vi "Update Channel UI.vi"(8 "error in (no error)":errorcluster, 10 "Channels":T1[][](array[typedef]), 11 "CIF_UI in":refnum<class "CIF_UI.lvclass">) -> (0 "error out":errorcluster, 3 "CIF_UI out":refnum<class "CIF_UI.lvclass">)   [LabVIEW 2021, in "CIF_UI.lvclass"]
uses:
  CIF_UI.lvclass
  CIFCore/Grpc/CIFCoreChannel_client/RPC Messages/cif_channelcore_Channel.ctl
  CIFCore/Grpc/CIFCoreChannel_client/RPC Messages/cif_channelcore_Direction.ctl
  CIFCore/Grpc/CIFCoreChannel_client/RPC Messages/cif_channelcore_PATTERN.ctl
  CIF_UI.lvclass/CIF_UI.ctl
  Typedef/Direction to Include.ctl
  CIFCore/Grpc/CIFCoreChannel_client/CIFCoreChannel_client.lvlib
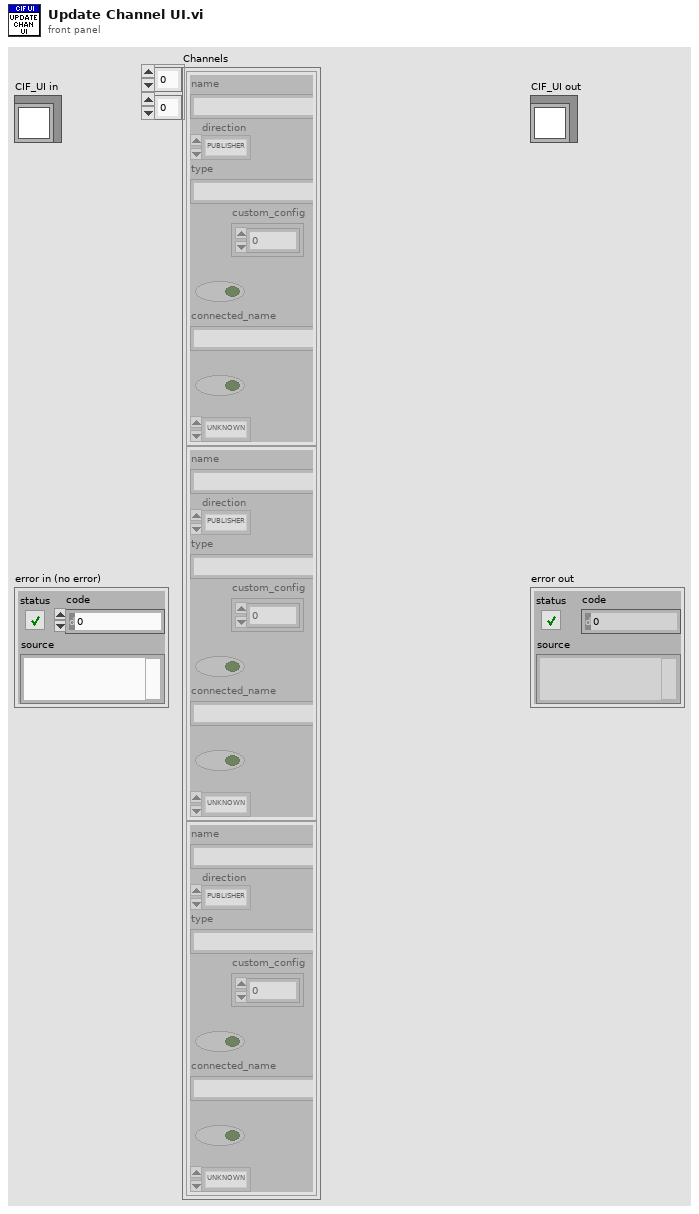
[diagram p1: front panel]
types:
  T1 = typedef "CIFCoreChannel_client.lvlib/cif_channelcore_Channel.ctl" = cluster{"name":string, "direction":T2, "type":string, "custom_config":u8[], "connected":bool, "connected_name":string, "forced":bool, "channel_pattern":T3}
  T2 = typedef "CIFCoreChannel_client.lvlib/cif_channelcore_Direction.ctl" = enum32{"PUBLISHER", "SUBSCRIBER"}
  T3 = typedef "CIFCoreChannel_client.lvlib/cif_channelcore_PATTERN.ctl" = enum32{"UNKNOWN", "TAG", "FIFO", "MULTIFIFO"}
  T4 = typedef "CIF_UI.lvclass/Direction to Include.ctl" = enum16{"All", "Subscriber", "Publisher"}
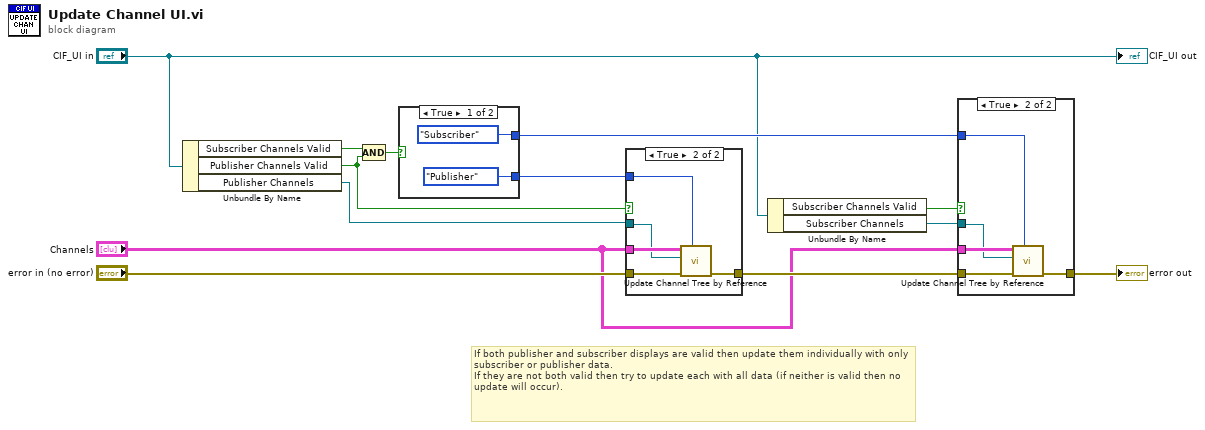
[diagram p0: block diagram]
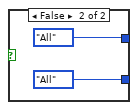
[diagram p2: hidden frame]
diagram:
  # "If both publisher and subscriber displays are valid then update them individually with only subscriber or publisher data.  \nIf they are not both valid then try to update each with all data (if neither is valid then no update will occur)."
  n1 = Unbundle By Name("CIF_UI in") -> ("Subscriber Channels Valid"=w13:bool, "Publisher Channels Valid"=w4:bool, "Publisher Channels"=w3:refnum<vi>)
  n2 = Compound Arithmetic op=AND(w13, w4) -> (w7:bool)
  n3 = case shown="True" w7 {
    tunnel: [Direction_to_Include."Subscriber" ("Direction to Include") Direction_to_Include."All" ("Direction to Include")] -> w5
    tunnel: [Direction_to_Include."Publisher" ("Direction to Include") Direction_to_Include."All" ("Direction to Include")] -> w6
    frame True {
    }
    frame False {
    }
  }
  n4 = case shown="True" w4 {
    tunnel: "Channels" -> [_ w23]
    tunnel: w3 -> [_ w22]
    tunnel: w6 -> [_ w21]
    tunnel: "error in (no error)" -> [w18 w20]
    tunnel: [w18 w19] -> w10
    frame False {
    }
    frame True {
      n5 = call "Update Channel Tree by Reference.vi"("Direction to Include"=w21, "error in (no error)"=w20, "Channnel Tree ref in"=w22, "Channels"=w23) -> ("error out"=w19:errorcluster)  [unwired: 7 in]
    }
  }
  n6 = Unbundle By Name("CIF_UI in") -> ("Subscriber Channels Valid"=w11:bool, "Subscriber Channels"=w12:refnum<vi>)
  n7 = case shown="True" w11 {
    tunnel: "Channels" -> [_ w29]
    tunnel: w12 -> [_ w28]
    tunnel: w5 -> [_ w27]
    tunnel: w10 -> [w24 w26]
    tunnel: [w24 w25] -> w8
    frame False {
    }
    frame True {
      n8 = call "Update Channel Tree by Reference.vi"("Direction to Include"=w27, "error in (no error)"=w26, "Channnel Tree ref in"=w28, "Channels"=w29) -> ("error out"=w25:errorcluster)  [unwired: 7 in]
    }
  }
  "error out" <- w8
  "CIF_UI out" <- "CIF_UI in"
